vi "Delete Uint32 DVR.vi"(8 "error in (no error)":errorcluster, 11 "Uint32 DVR in":refnum<data-value>) -> (0 "error out":errorcluster, 3 "Uint32 out":refnum<class "Uint32.lvclass">)   [LabVIEW 2015, in "MDSplus.lvlib" / "Uint32.lvclass"]
uses:
  Uint32.lvclass
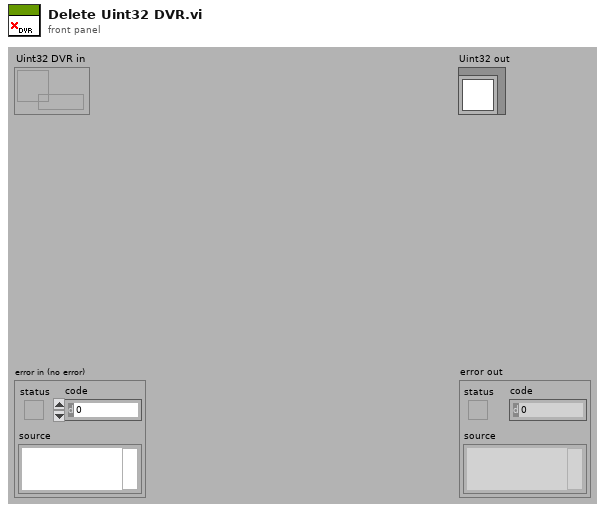
[diagram p1: front panel]
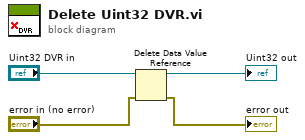
[diagram p0: block diagram]
diagram:
  n1 = Delete Data Value Reference(data value reference="Uint32 DVR in", error in="error in (no error)") -> (data value=→"Uint32 out":refnum<class "Uint32.lvclass">, error out=→"error out":errorcluster)
